vi "dispatcher.vi"() -> ()   [LabVIEW 2025]
panel:
  out "status":string
  out "time":dbl format="%.3f"
  out "time stamp":timestamp
  in  "reading":T1
  in  "writing":T2
  in  "vi path":path=path "H:/LabVIEW/_python control/demo target.vi"
  in  "stop":bool
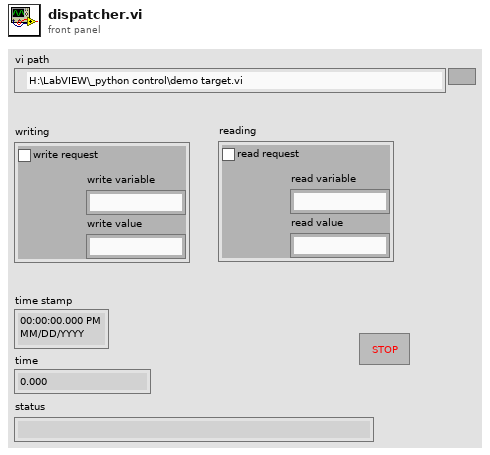
[diagram p1: front panel]
types:
  T1 = cluster{"read request":bool, "read variable":string, "read value":string}
  T2 = cluster{"write request":bool, "write variable":string, "write value":string}
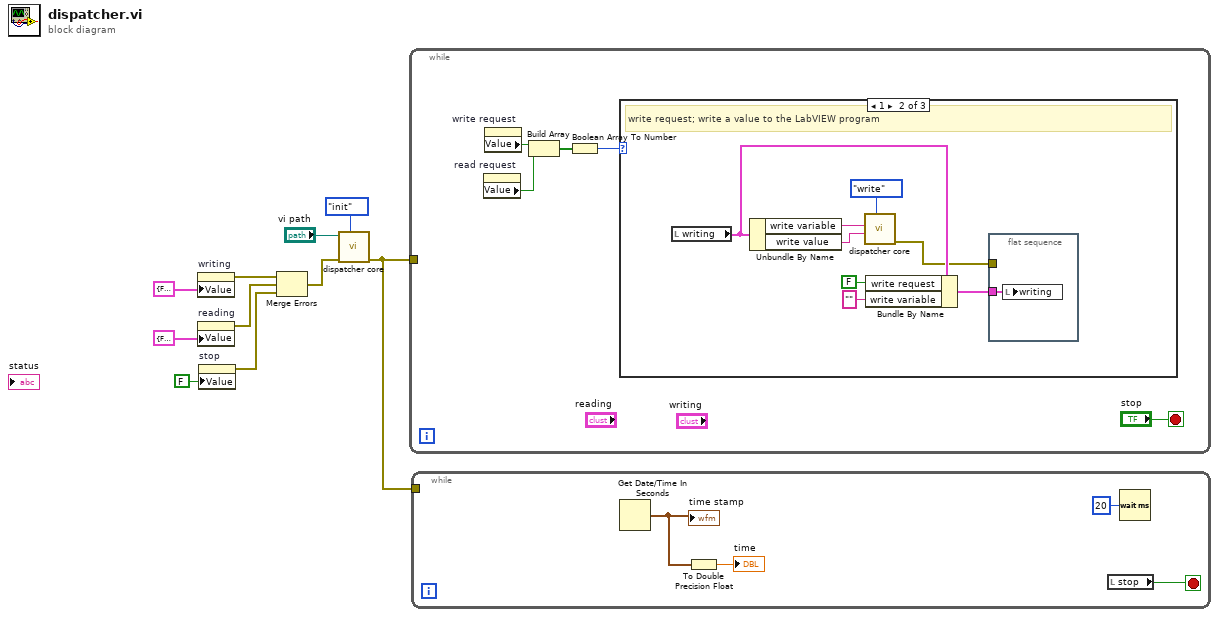
[diagram p0: block diagram]
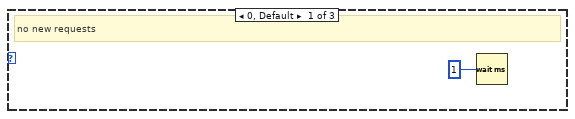
[diagram p2: hidden frame]
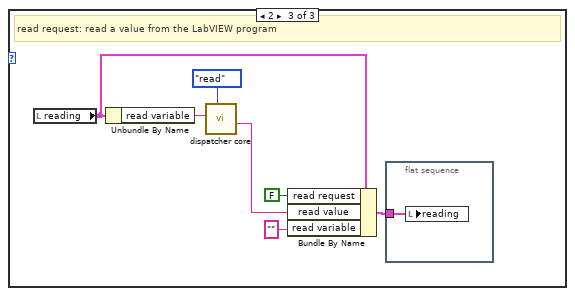
[diagram p3: hidden frame]
diagram:
  n1 = property on="writing" class="Clust (strict)"("Value"=T2 {"write request"=FALSE, "write variable"="", "write value"=""} ("writing")) -> (error out=w6:errorcluster)  [unwired: 2 in, 1 out]
  n2 = property on="reading" class="Clust (strict)"("Value"=T2 {"write request"=FALSE, "write variable"="", "write value"=""} ("writing")) -> (error out=w5:errorcluster)  [unwired: 2 in, 1 out]
  n3 = property on="stop" class="Bool (strict)"("Value"=FALSE ("stop")) -> (error out=w2:errorcluster)  [unwired: 2 in, 1 out]
  n4 = Merge Errors(w6, w5, w2) -> (w4:errorcluster)
  n5 = call "dispatcher core.vi"("action"=enum16{"init", "read", "write"}."init", "error in (no error)"=w4, "vi path"="vi path") -> ("error out"=w1:errorcluster)  [unwired: 7 in, 1 out]
  n6 = while {
    tunnel: w1 -> [_]
    stop <- "stop" stop-if-true
    n7 = property on="read request" class="Bool (strict)"() -> ("Value"=w13:bool)  [unwired: 2 in, 2 out]
    n8 = property on="write request" class="Bool (strict)"() -> ("Value"=w14:bool)  [unwired: 2 in, 2 out]
    n9 = Build Array(w14, w13) -> (w12:bool[])
    n10 = Boolean Array To Number(Boolean array=w12) -> (number=w11:u8)
    n11 = case shown="1" w11 {
      frame 0, Default {
        # "no new requests"
        n12 = Wait (ms)(milliseconds to wait=u32 1) -> ()  [unwired: 1 out]
      }
      frame 1 {
        # "write request; write a value to the LabVIEW program"
        n13 = local read "writing"() -> (w21:T2)
        n14 = Unbundle By Name(w21) -> ("write variable"=w23:string, "write value"=w22:string)
        n15 = call "dispatcher core.vi"("action"=enum16{"init", "read", "write"}."write", "control value (in)"=w22, "control name"=w23) -> ("error out"=w17:errorcluster)  [unwired: 7 in, 1 out]
        n16 = Bundle By Name(cluster=w21, "write request"=FALSE, "write variable"="") -> (w18:T2)
        n17 = flat-sequence {
          tunnel: w18 -> [w25]
          tunnel: w17 -> [_]
          frame #0 {
            n18 = local write "writing"(w25) -> ()
          }
        }
      }
      frame 2 {
        # "read request: read a value from the LabVIEW program"
        n19 = local read "reading"() -> (w30:T1)
        n20 = Unbundle By Name(w30) -> ("read variable"=w31:string)
        n21 = call "dispatcher core.vi"("action"=enum16{"init", "read", "write"}."read", "control name"=w31) -> ("control value (out)"=w28:string)  [unwired: 8 in, 1 out]
        n22 = Bundle By Name(cluster=w30, "read request"=FALSE, "read value"=w28, "read variable"="") -> (w27:T1)
        n23 = flat-sequence {
          tunnel: w27 -> [w33]
          frame #0 {
            n24 = local write "reading"(w33) -> ()
          }
        }
      }
    }
  }
  n25 = while {
    tunnel: w1 -> [_]
    stop <- w37 stop-if-true
    n26 = Get Date/Time In Seconds() -> (seconds since 1Jan1904=w35:timestamp)
    "time stamp" <- w35
    n27 = To Double Precision Float(number=w35) -> (double precision float=→"time":dbl)
    n28 = local read "stop"() -> (w37:bool)
    n29 = Wait (ms)(milliseconds to wait=u32 20) -> ()  [unwired: 1 out]
  }
